vi "maxwell.vi"() -> ()   [LabVIEW 2011]
panel:
  out "LILLY MATAH BUFF TURNS":i32
  in  "OK Button":bool
  out "turn 20":bool
  out "turn 19":bool
  out "turn 18":bool
  out "turn 17":bool
  out "turn 16":bool
  out "turn 15":bool
  out "turn 14":bool
  out "turn 13":bool
  out "turn 12":bool
  out "turn 11":bool
  out "turn 10":bool
  out "turn 9":bool
  out "turn 8":bool
  out "turn 7":bool
  out "turn 6":bool
  out "turn 5":bool
  out "turn 4":bool
  out "turn 3":bool
  out "turn 2":bool
  in  "stop":bool
  out "turn 1":bool
  in  "Turns":i32=1 min=1 max=21
  # "IGNORE DEF"
  # "MATAH BB"
  # "GUARD"
  # "SS1"
  # "SS2"
  # "RUNE"
  # "IGNORE DEF"
  # "MATAH BB"
  # "GUARD"
  # "SS2"
  # "SS1"
  # "DESTINY"
  # "RUNE"
  # "IGNORE DEF"
  # "MATAH BB"
  # "GUARD"
  # "SS1"
  # "SS2"
  # "DESTINY"
  # "RUNE"
  # "MATAH BB"
  # "GUARD"
  # "IGNORE DEF"
  # "SS1"
  # "SS2"
  # "DESTINY"
  # "RUNE"
  # "IGNORE DEF"
  # "MATAH BB"
  # "GUARD"
  # "SS1"
  # "SS2"
  # "RUNE,DESTINY"
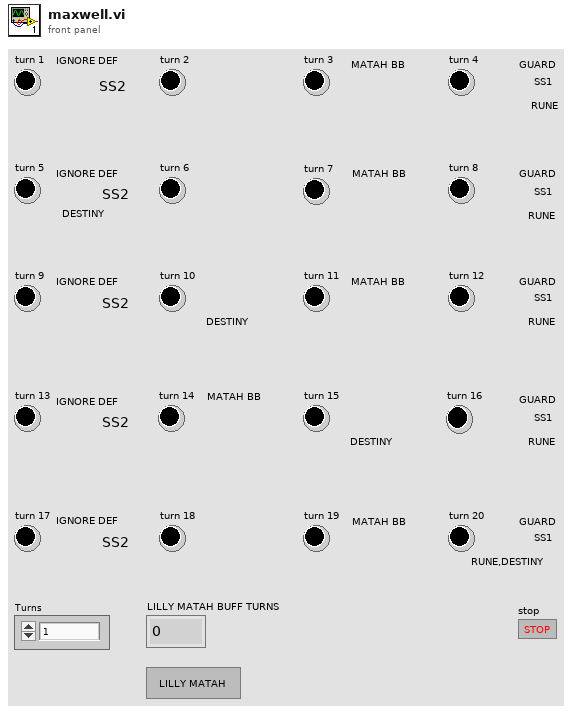
[diagram p1: front panel]
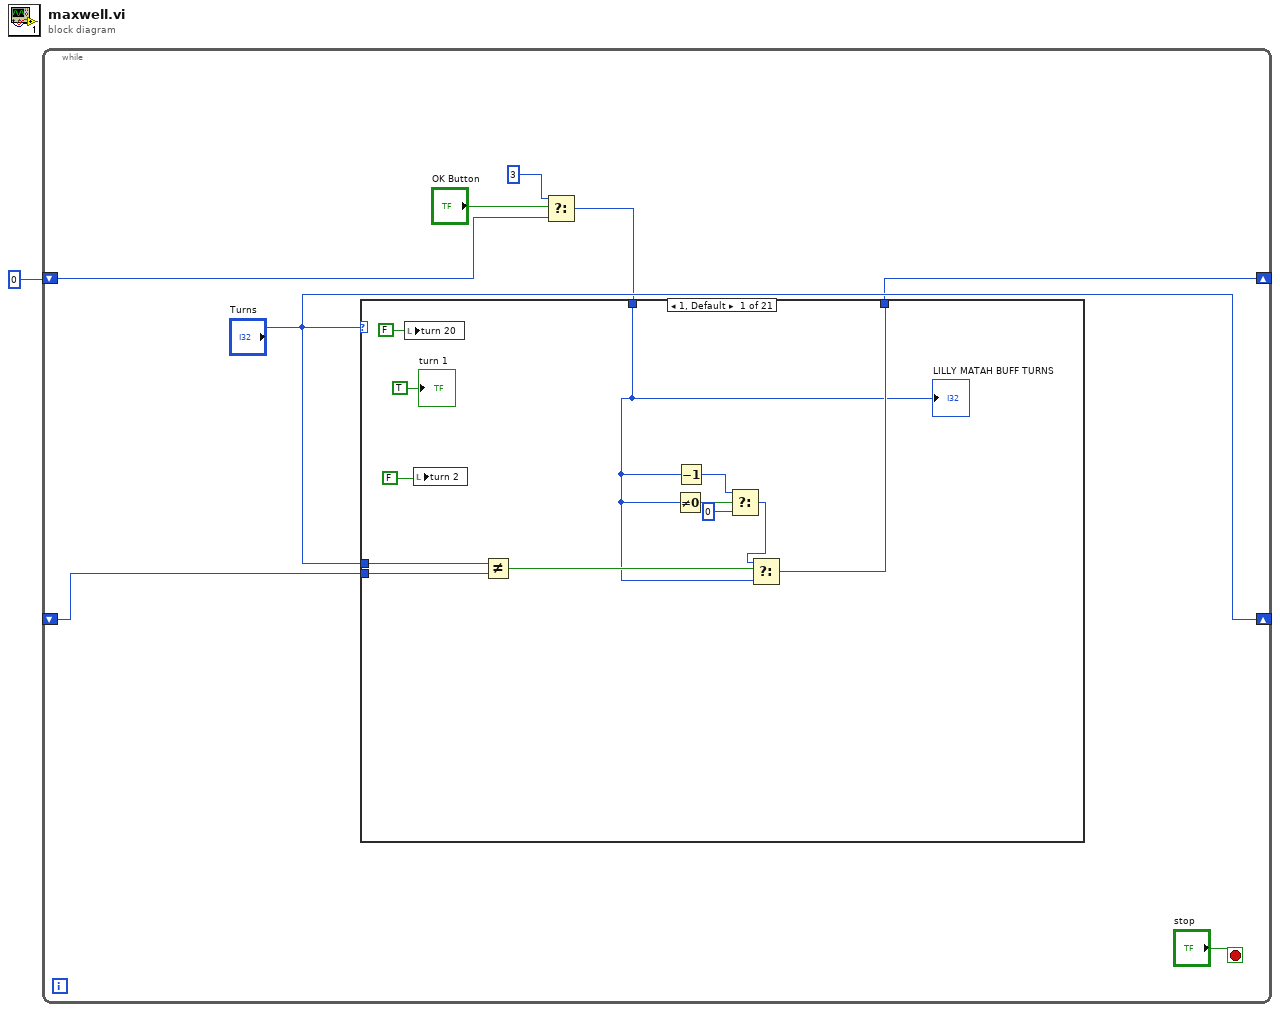
[diagram p0: block diagram]
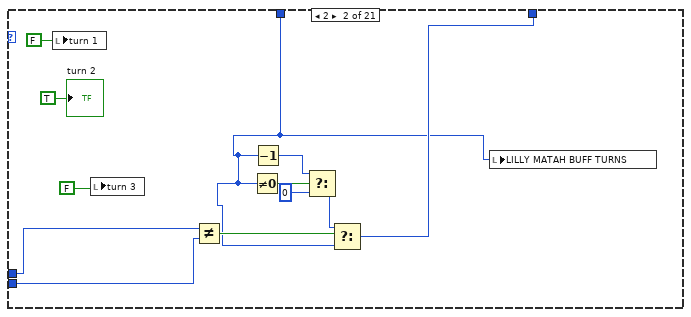
[diagram p2: hidden frame]
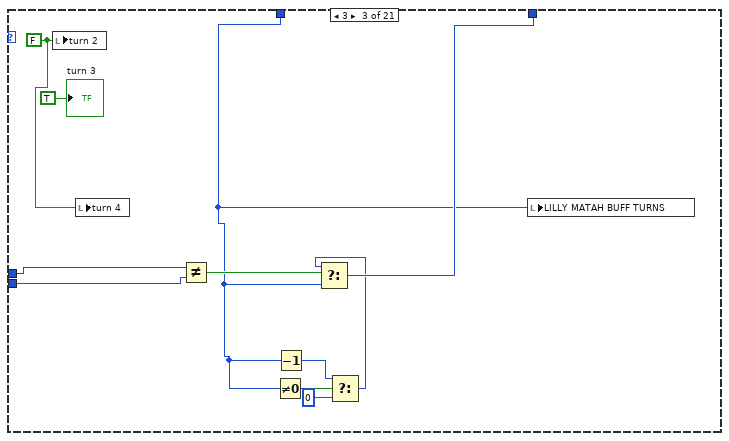
[diagram p3: hidden frame]
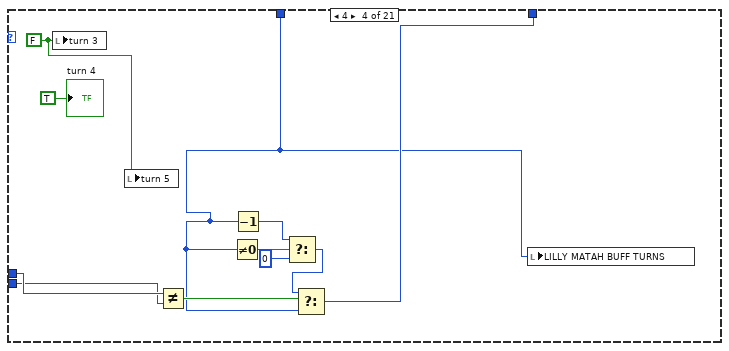
[diagram p4: hidden frame]
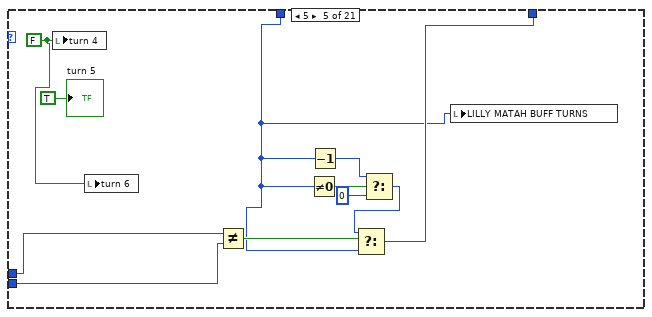
[diagram p5: hidden frame]
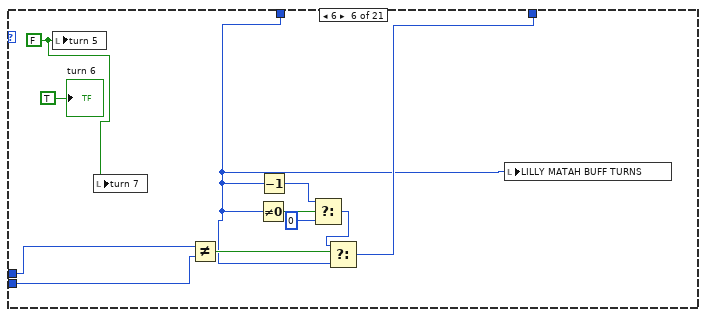
[diagram p6: hidden frame]
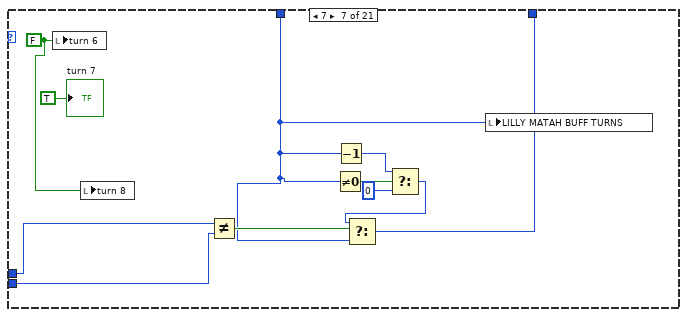
[diagram p7: hidden frame]
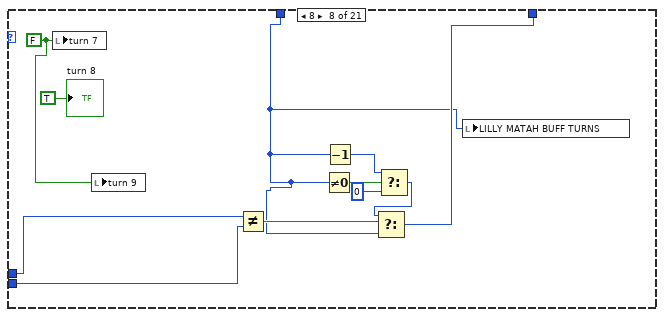
[diagram p8: hidden frame]
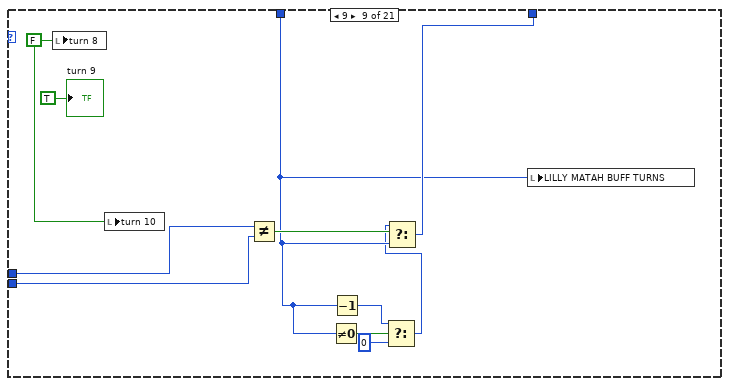
[diagram p9: hidden frame]
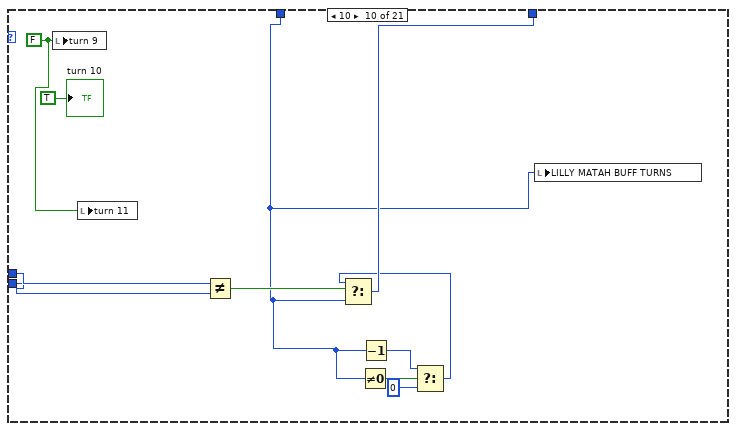
[diagram p10: hidden frame]
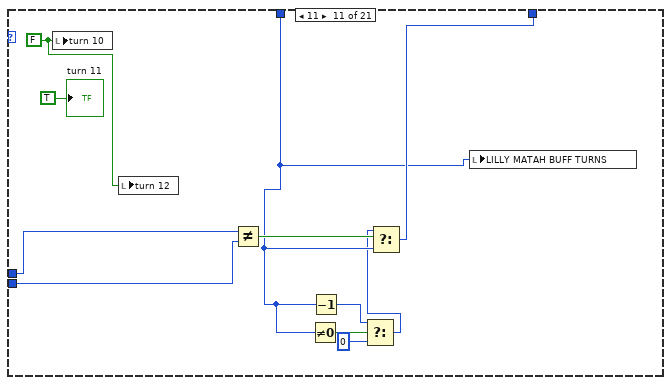
[diagram p11: hidden frame]
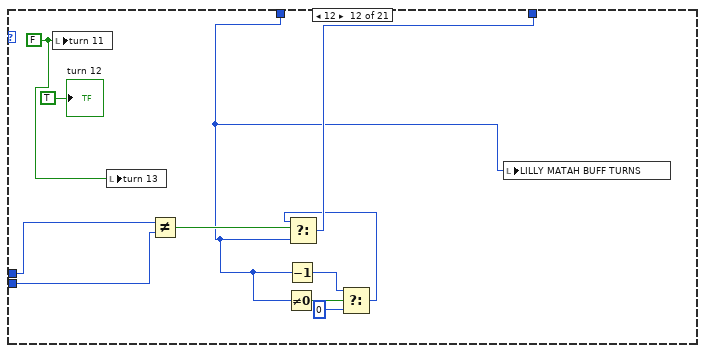
[diagram p12: hidden frame]
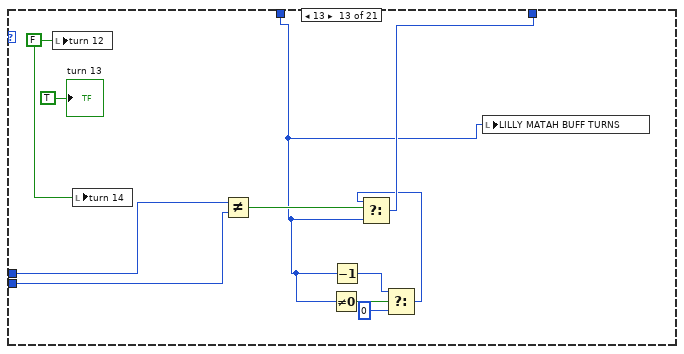
[diagram p13: hidden frame]
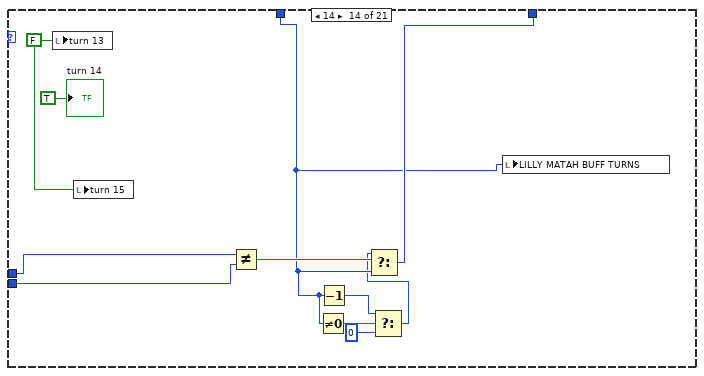
[diagram p14: hidden frame]
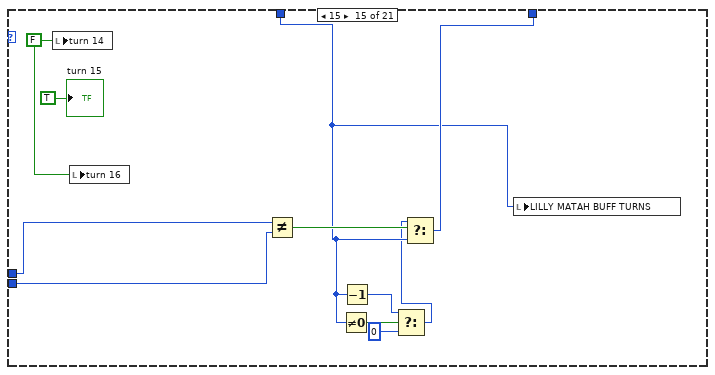
[diagram p15: hidden frame]
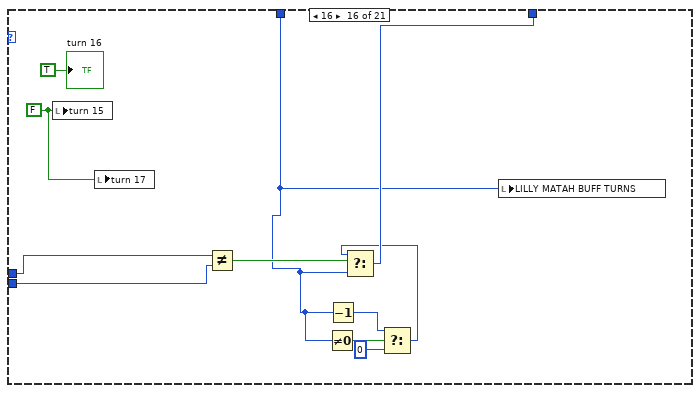
[diagram p16: hidden frame]
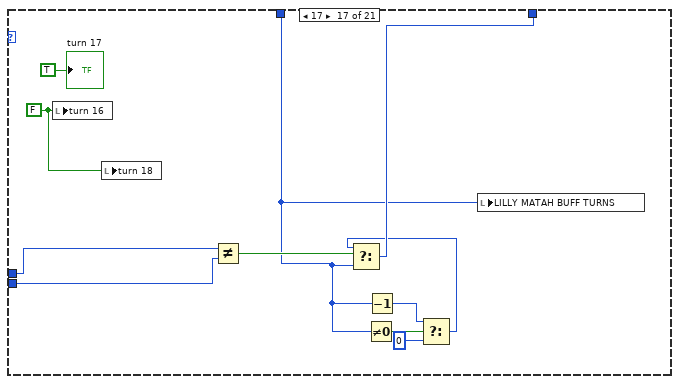
[diagram p17: hidden frame]
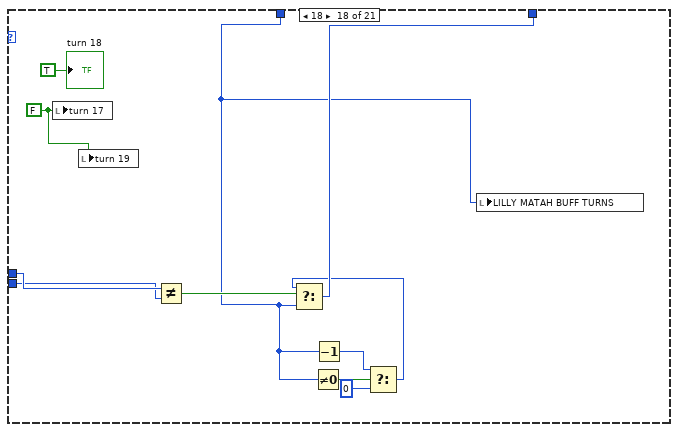
[diagram p18: hidden frame]
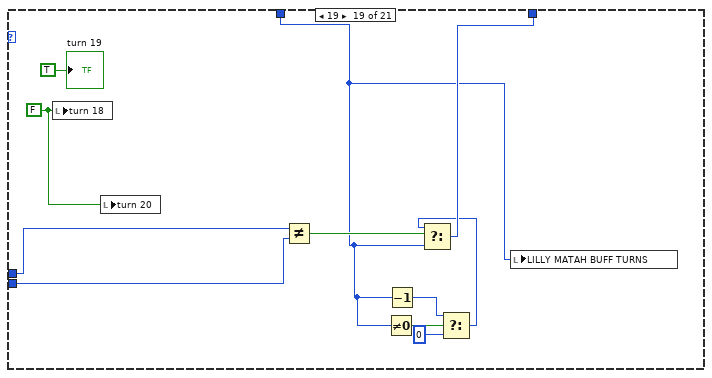
[diagram p19: hidden frame]
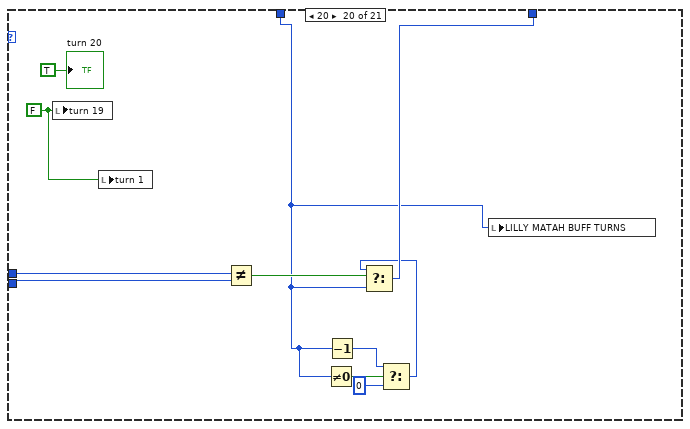
[diagram p20: hidden frame]
diagram:
  n1 = while {
    shift-right: [w2] -> _
    shift-left: 0 -> [w4]
    shift-right: ["Turns"] -> _
    shift-left: _ -> [w7]
    stop <- "stop" stop-if-true
    n2 = Select(t=3, s="OK Button", f=w4) -> (s? t:f=w3:i32)
    n3 = case shown="1, Default" "Turns" {
      tunnel: w3 -> [w14 w23 w35 w46 w57 w68 w79 w90 w101 w112 w123 w134 w145 w156 w167 w178 w189 w200 w211 w222 w232]
      tunnel: [w15 w27 w39 w50 w61 w72 w83 w94 w105 w116 w127 w138 w149 w160 w171 w182 w193 w204 w215 w226 w232] -> w2
      tunnel: "Turns" -> [w18 w29 w41 w52 w63 w74 w85 w96 w107 w118 w129 w140 w151 w162 w173 w184 w195 w206 w217 w228 _]
      tunnel: w7 -> [w17 w28 w40 w51 w62 w73 w84 w95 w106 w117 w128 w139 w150 w161 w172 w183 w194 w205 w216 w227 _]
      frame 1, Default {
        n4 = local write "turn 20"(FALSE ("Boolean")) -> ()
        n5 = local write "turn 2"(FALSE ("Boolean")) -> ()
        n6 = Not Equal?(x=w18, y=w17) -> (x != y?=w16:bool)
        n7 = Not Equal To 0?(x=w14) -> (x != 0?=w13:bool)
        n8 = Decrement(x=w14) -> (x-1=w12:i32)
        n9 = Select(t=w12, s=w13, f=0) -> (s? t:f=w10:i32)
        n10 = Select(t=w10, s=w16, f=w14) -> (s? t:f=w15:i32)
        "turn 1" <- TRUE ("Boolean")
        "LILLY MATAH BUFF TURNS" <- w14
      }
      frame 2 {
        n11 = local write "turn 1"(FALSE ("turn 1")) -> ()
        n12 = local write "turn 3"(FALSE ("turn 1")) -> ()
        n13 = Not Equal?(x=w29, y=w28) -> (x != y?=w30:bool)
        n14 = Not Equal To 0?(x=w23) -> (x != 0?=w26:bool)
        n15 = Decrement(x=w23) -> (x-1=w25:i32)
        n16 = Select(t=w25, s=w26, f=0) -> (s? t:f=w22:i32)
        n17 = Select(t=w22, s=w30, f=w23) -> (s? t:f=w27:i32)
        n18 = local write "LILLY MATAH BUFF TURNS"(w23) -> ()
        "turn 2" <- TRUE ("turn 2")
      }
      frame 3 {
        w43 = FALSE ("turn 2")
        n19 = local write "turn 2"(w43) -> ()
        n20 = local write "turn 4"(w43) -> ()
        n21 = Not Equal?(x=w41, y=w40) -> (x != y?=w42:bool)
        n22 = Not Equal To 0?(x=w35) -> (x != 0?=w38:bool)
        n23 = Decrement(x=w35) -> (x-1=w37:i32)
        n24 = Select(t=w37, s=w38, f=0) -> (s? t:f=w34:i32)
        n25 = Select(t=w34, s=w42, f=w35) -> (s? t:f=w39:i32)
        n26 = local write "LILLY MATAH BUFF TURNS"(w35) -> ()
        "turn 3" <- TRUE ("turn 3")
      }
      frame 4 {
        w54 = FALSE ("turn 1")
        n27 = local write "turn 3"(w54) -> ()
        n28 = local write "turn 5"(w54) -> ()
        n29 = Not Equal?(x=w52, y=w51) -> (x != y?=w53:bool)
        n30 = Not Equal To 0?(x=w46) -> (x != 0?=w49:bool)
        n31 = Decrement(x=w46) -> (x-1=w48:i32)
        n32 = Select(t=w48, s=w49, f=0) -> (s? t:f=w45:i32)
        n33 = Select(t=w45, s=w53, f=w46) -> (s? t:f=w50:i32)
        n34 = local write "LILLY MATAH BUFF TURNS"(w46) -> ()
        "turn 4" <- TRUE ("turn 2")
      }
      frame 5 {
        w65 = FALSE ("turn 1")
        n35 = local write "turn 4"(w65) -> ()
        n36 = local write "turn 6"(w65) -> ()
        n37 = Not Equal?(x=w63, y=w62) -> (x != y?=w64:bool)
        n38 = Not Equal To 0?(x=w57) -> (x != 0?=w60:bool)
        n39 = Decrement(x=w57) -> (x-1=w59:i32)
        n40 = Select(t=w59, s=w60, f=0) -> (s? t:f=w56:i32)
        n41 = Select(t=w56, s=w64, f=w57) -> (s? t:f=w61:i32)
        n42 = local write "LILLY MATAH BUFF TURNS"(w57) -> ()
        "turn 5" <- TRUE ("turn 2")
      }
      frame 6 {
        w76 = FALSE ("turn 1")
        n43 = local write "turn 5"(w76) -> ()
        n44 = local write "turn 7"(w76) -> ()
        n45 = Not Equal?(x=w74, y=w73) -> (x != y?=w75:bool)
        n46 = Not Equal To 0?(x=w68) -> (x != 0?=w71:bool)
        n47 = Decrement(x=w68) -> (x-1=w70:i32)
        n48 = Select(t=w70, s=w71, f=0) -> (s? t:f=w67:i32)
        n49 = Select(t=w67, s=w75, f=w68) -> (s? t:f=w72:i32)
        n50 = local write "LILLY MATAH BUFF TURNS"(w68) -> ()
        "turn 6" <- TRUE ("turn 2")
      }
      frame 7 {
        w87 = FALSE ("turn 1")
        n51 = local write "turn 6"(w87) -> ()
        n52 = local write "turn 8"(w87) -> ()
        n53 = Not Equal?(x=w85, y=w84) -> (x != y?=w86:bool)
        n54 = Not Equal To 0?(x=w79) -> (x != 0?=w82:bool)
        n55 = Decrement(x=w79) -> (x-1=w81:i32)
        n56 = Select(t=w81, s=w82, f=0) -> (s? t:f=w78:i32)
        n57 = Select(t=w78, s=w86, f=w79) -> (s? t:f=w83:i32)
        n58 = local write "LILLY MATAH BUFF TURNS"(w79) -> ()
        "turn 7" <- TRUE ("turn 2")
      }
      frame 8 {
        w98 = FALSE ("turn 1")
        n59 = local write "turn 7"(w98) -> ()
        n60 = local write "turn 9"(w98) -> ()
        n61 = Not Equal?(x=w96, y=w95) -> (x != y?=w97:bool)
        n62 = Not Equal To 0?(x=w90) -> (x != 0?=w93:bool)
        n63 = Decrement(x=w90) -> (x-1=w92:i32)
        n64 = Select(t=w92, s=w93, f=0) -> (s? t:f=w89:i32)
        n65 = Select(t=w89, s=w97, f=w90) -> (s? t:f=w94:i32)
        n66 = local write "LILLY MATAH BUFF TURNS"(w90) -> ()
        "turn 8" <- TRUE ("turn 2")
      }
      frame 9 {
        w109 = FALSE ("turn 1")
        n67 = local write "turn 8"(w109) -> ()
        n68 = local write "turn 10"(w109) -> ()
        n69 = Not Equal?(x=w107, y=w106) -> (x != y?=w108:bool)
        n70 = Not Equal To 0?(x=w101) -> (x != 0?=w104:bool)
        n71 = Decrement(x=w101) -> (x-1=w103:i32)
        n72 = Select(t=w103, s=w104, f=0) -> (s? t:f=w100:i32)
        n73 = Select(t=w100, s=w108, f=w101) -> (s? t:f=w105:i32)
        n74 = local write "LILLY MATAH BUFF TURNS"(w101) -> ()
        "turn 9" <- TRUE ("turn 2")
      }
      frame 10 {
        w120 = FALSE ("turn 1")
        n75 = local write "turn 9"(w120) -> ()
        n76 = local write "turn 11"(w120) -> ()
        n77 = Not Equal?(x=w118, y=w117) -> (x != y?=w119:bool)
        n78 = Not Equal To 0?(x=w112) -> (x != 0?=w115:bool)
        n79 = Decrement(x=w112) -> (x-1=w114:i32)
        n80 = Select(t=w114, s=w115, f=0) -> (s? t:f=w111:i32)
        n81 = Select(t=w111, s=w119, f=w112) -> (s? t:f=w116:i32)
        n82 = local write "LILLY MATAH BUFF TURNS"(w112) -> ()
        "turn 10" <- TRUE ("turn 2")
      }
      frame 11 {
        w131 = FALSE ("turn 1")
        n83 = local write "turn 10"(w131) -> ()
        n84 = local write "turn 12"(w131) -> ()
        n85 = Not Equal?(x=w129, y=w128) -> (x != y?=w130:bool)
        n86 = Not Equal To 0?(x=w123) -> (x != 0?=w126:bool)
        n87 = Decrement(x=w123) -> (x-1=w125:i32)
        n88 = Select(t=w125, s=w126, f=0) -> (s? t:f=w122:i32)
        n89 = Select(t=w122, s=w130, f=w123) -> (s? t:f=w127:i32)
        n90 = local write "LILLY MATAH BUFF TURNS"(w123) -> ()
        "turn 11" <- TRUE ("turn 2")
      }
      frame 12 {
        w142 = FALSE ("turn 1")
        n91 = local write "turn 11"(w142) -> ()
        n92 = local write "turn 13"(w142) -> ()
        n93 = Not Equal?(x=w140, y=w139) -> (x != y?=w141:bool)
        n94 = Not Equal To 0?(x=w134) -> (x != 0?=w137:bool)
        n95 = Decrement(x=w134) -> (x-1=w136:i32)
        n96 = Select(t=w136, s=w137, f=0) -> (s? t:f=w133:i32)
        n97 = Select(t=w133, s=w141, f=w134) -> (s? t:f=w138:i32)
        n98 = local write "LILLY MATAH BUFF TURNS"(w134) -> ()
        "turn 12" <- TRUE ("turn 2")
      }
      frame 13 {
        w153 = FALSE ("turn 1")
        n99 = local write "turn 12"(w153) -> ()
        n100 = local write "turn 14"(w153) -> ()
        n101 = Not Equal?(x=w151, y=w150) -> (x != y?=w152:bool)
        n102 = Not Equal To 0?(x=w145) -> (x != 0?=w148:bool)
        n103 = Decrement(x=w145) -> (x-1=w147:i32)
        n104 = Select(t=w147, s=w148, f=0) -> (s? t:f=w144:i32)
        n105 = Select(t=w144, s=w152, f=w145) -> (s? t:f=w149:i32)
        n106 = local write "LILLY MATAH BUFF TURNS"(w145) -> ()
        "turn 13" <- TRUE ("turn 2")
      }
      frame 14 {
        w164 = FALSE ("turn 1")
        n107 = local write "turn 13"(w164) -> ()
        n108 = local write "turn 15"(w164) -> ()
        n109 = Not Equal?(x=w162, y=w161) -> (x != y?=w163:bool)
        n110 = Not Equal To 0?(x=w156) -> (x != 0?=w159:bool)
        n111 = Decrement(x=w156) -> (x-1=w158:i32)
        n112 = Select(t=w158, s=w159, f=0) -> (s? t:f=w155:i32)
        n113 = Select(t=w155, s=w163, f=w156) -> (s? t:f=w160:i32)
        n114 = local write "LILLY MATAH BUFF TURNS"(w156) -> ()
        "turn 14" <- TRUE ("turn 2")
      }
      frame 15 {
        w175 = FALSE ("turn 1")
        n115 = local write "turn 14"(w175) -> ()
        n116 = local write "turn 16"(w175) -> ()
        n117 = Not Equal?(x=w173, y=w172) -> (x != y?=w174:bool)
        n118 = Not Equal To 0?(x=w167) -> (x != 0?=w170:bool)
        n119 = Decrement(x=w167) -> (x-1=w169:i32)
        n120 = Select(t=w169, s=w170, f=0) -> (s? t:f=w166:i32)
        n121 = Select(t=w166, s=w174, f=w167) -> (s? t:f=w171:i32)
        n122 = local write "LILLY MATAH BUFF TURNS"(w167) -> ()
        "turn 15" <- TRUE ("turn 2")
      }
      frame 16 {
        w186 = FALSE ("turn 1")
        n123 = local write "turn 15"(w186) -> ()
        n124 = local write "turn 17"(w186) -> ()
        n125 = Not Equal?(x=w184, y=w183) -> (x != y?=w185:bool)
        n126 = Not Equal To 0?(x=w178) -> (x != 0?=w181:bool)
        n127 = Decrement(x=w178) -> (x-1=w180:i32)
        n128 = Select(t=w180, s=w181, f=0) -> (s? t:f=w177:i32)
        n129 = Select(t=w177, s=w185, f=w178) -> (s? t:f=w182:i32)
        n130 = local write "LILLY MATAH BUFF TURNS"(w178) -> ()
        "turn 16" <- TRUE ("turn 2")
      }
      frame 17 {
        w197 = FALSE ("turn 1")
        n131 = local write "turn 16"(w197) -> ()
        n132 = local write "turn 18"(w197) -> ()
        n133 = Not Equal?(x=w195, y=w194) -> (x != y?=w196:bool)
        n134 = Not Equal To 0?(x=w189) -> (x != 0?=w192:bool)
        n135 = Decrement(x=w189) -> (x-1=w191:i32)
        n136 = Select(t=w191, s=w192, f=0) -> (s? t:f=w188:i32)
        n137 = Select(t=w188, s=w196, f=w189) -> (s? t:f=w193:i32)
        n138 = local write "LILLY MATAH BUFF TURNS"(w189) -> ()
        "turn 17" <- TRUE ("turn 2")
      }
      frame 18 {
        w208 = FALSE ("turn 1")
        n139 = local write "turn 17"(w208) -> ()
        n140 = local write "turn 19"(w208) -> ()
        n141 = Not Equal?(x=w206, y=w205) -> (x != y?=w207:bool)
        n142 = Not Equal To 0?(x=w200) -> (x != 0?=w203:bool)
        n143 = Decrement(x=w200) -> (x-1=w202:i32)
        n144 = Select(t=w202, s=w203, f=0) -> (s? t:f=w199:i32)
        n145 = Select(t=w199, s=w207, f=w200) -> (s? t:f=w204:i32)
        n146 = local write "LILLY MATAH BUFF TURNS"(w200) -> ()
        "turn 18" <- TRUE ("turn 2")
      }
      frame 19 {
        w219 = FALSE ("turn 1")
        n147 = local write "turn 18"(w219) -> ()
        n148 = local write "turn 20"(w219) -> ()
        n149 = Not Equal?(x=w217, y=w216) -> (x != y?=w218:bool)
        n150 = Not Equal To 0?(x=w211) -> (x != 0?=w214:bool)
        n151 = Decrement(x=w211) -> (x-1=w213:i32)
        n152 = Select(t=w213, s=w214, f=0) -> (s? t:f=w210:i32)
        n153 = Select(t=w210, s=w218, f=w211) -> (s? t:f=w215:i32)
        n154 = local write "LILLY MATAH BUFF TURNS"(w211) -> ()
        "turn 19" <- TRUE ("turn 2")
      }
      frame 20 {
        w230 = FALSE ("turn 1")
        n155 = local write "turn 19"(w230) -> ()
        n156 = local write "turn 1"(w230) -> ()
        n157 = Not Equal?(x=w228, y=w227) -> (x != y?=w229:bool)
        n158 = Not Equal To 0?(x=w222) -> (x != 0?=w225:bool)
        n159 = Decrement(x=w222) -> (x-1=w224:i32)
        n160 = Select(t=w224, s=w225, f=0) -> (s? t:f=w221:i32)
        n161 = Select(t=w221, s=w229, f=w222) -> (s? t:f=w226:i32)
        n162 = local write "LILLY MATAH BUFF TURNS"(w222) -> ()
        "turn 20" <- TRUE ("turn 2")
      }
      frame 21 {
        n163 = invoke on="Turns" class="DigNum (strict)" method="Reinit To Default"() -> ()  [unwired: 3 in, 3 out]
      }
    }
  }
